vi "24.Evd.9_AskEfarmog.vi"() -> ()   [LabVIEW 2020]
uses:
  <vilib>/Native 3D Graph/xcontrol/3DPC_SurfacePlot.xctl
  <vilib>/measure/NI_MABase.lvlib
panel:
  in  "stop 3":bool
  out "Waveform Chart":waveform(dbl)[](graph)
  in  "Clear":bool
  in  "Boolean":bool
  in  "Boolean 2":bool
  in  "Boolean 3":bool
  in  "OK Button 4":bool
  in  "Frequency":dbl
  in  "Amplitude":dbl
  in  "stop 2":bool
  out "Waveform Graph":dbl[][](array[numeric])
  out "3D Graph":refnum<class "Base Datatype.lvclass">[](xcontrol)
  in  "OK Button 3":bool
  in  "Digital Data 2":digitaldata
  out "output waveform 2":digitalwaveform(waveform)={"t0"=timestamp(0 s since 1904-01-01), "dt"=1.0, "Y"={"transitions"=[], "data"=[]}}
  in  "stop":bool
  in  "OK Button 2":bool
  out "Digital Waveform Graph 3":digitalwaveform(graph)
  out "Digital Waveform Graph":digitalwaveform(graph)
  out "Sine Wave":waveform(dbl)[](graph)
  out "XY Graph":cluster{i32[], dbl[]}(graph)
  out "Random Array":dbl[](array[numeric])
  out "Waveform":waveform(dbl)[](graph)
  out "output waveform":digitalwaveform(waveform)={"t0"=timestamp(0 s since 1904-01-01), "dt"=1.0, "Y"={"transitions"=[], "data"=[]}}
  in  "Digital Data":digitaldata
  out "Mixed Signal Graph":T1(graph)
  out "Digital Waveform Graph 2":digitalwaveform(graph)
  in  "OK Button":bool
  # "11,33"
  # "11,35"
  # "11,39"
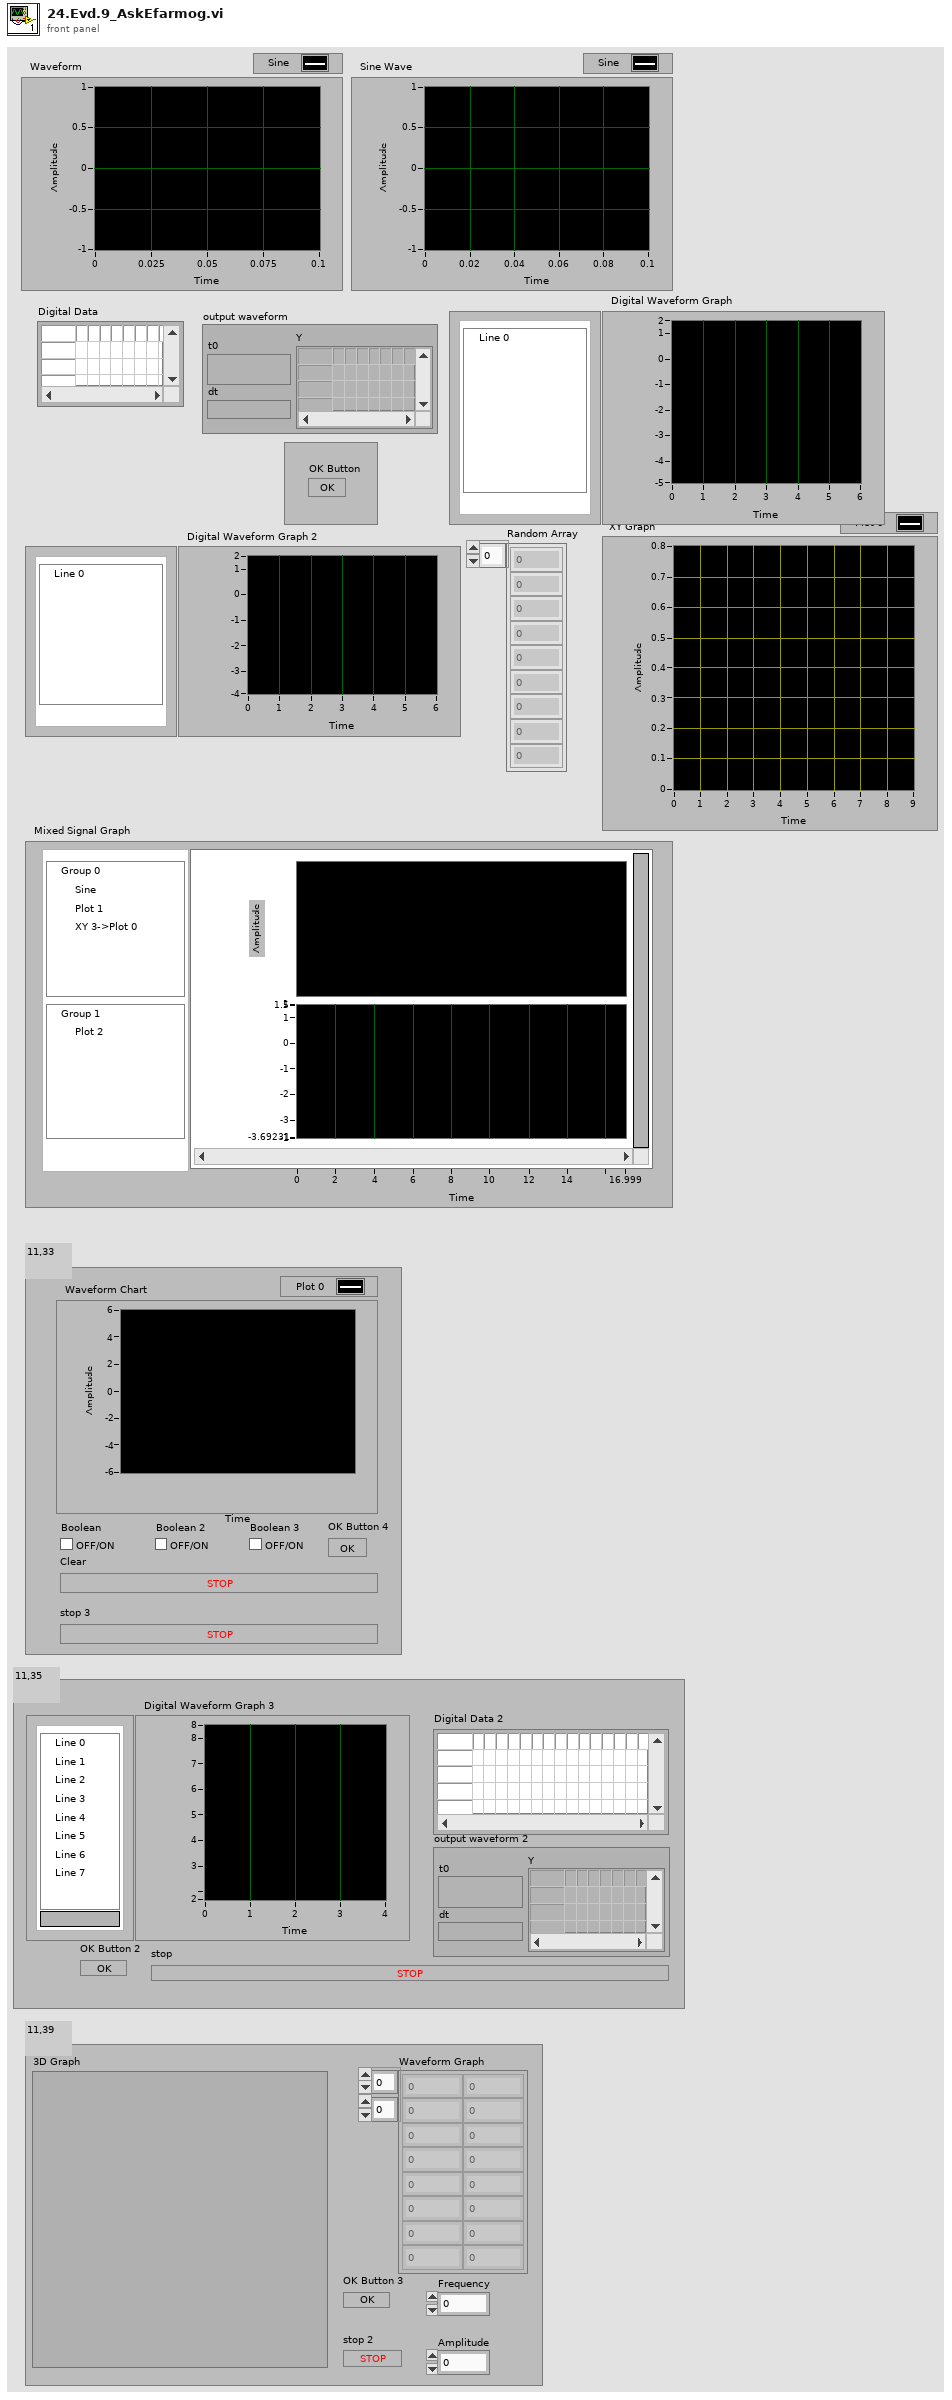
[diagram p1: front panel]
types:
  T1 = cluster{"Array of Waveform":waveform(dbl)[], dbl[], digitalwaveform, cluster{i32[], dbl[]}}
  T2 = typedef "imagedata.ctl" = cluster{"image type":i32, "image depth":i32, "image":u8[], "mask":u8[], "colors":u32[], "Rectangle":cluster{"left":i16, "top":i16, "right":i16, "bottom":i16}}
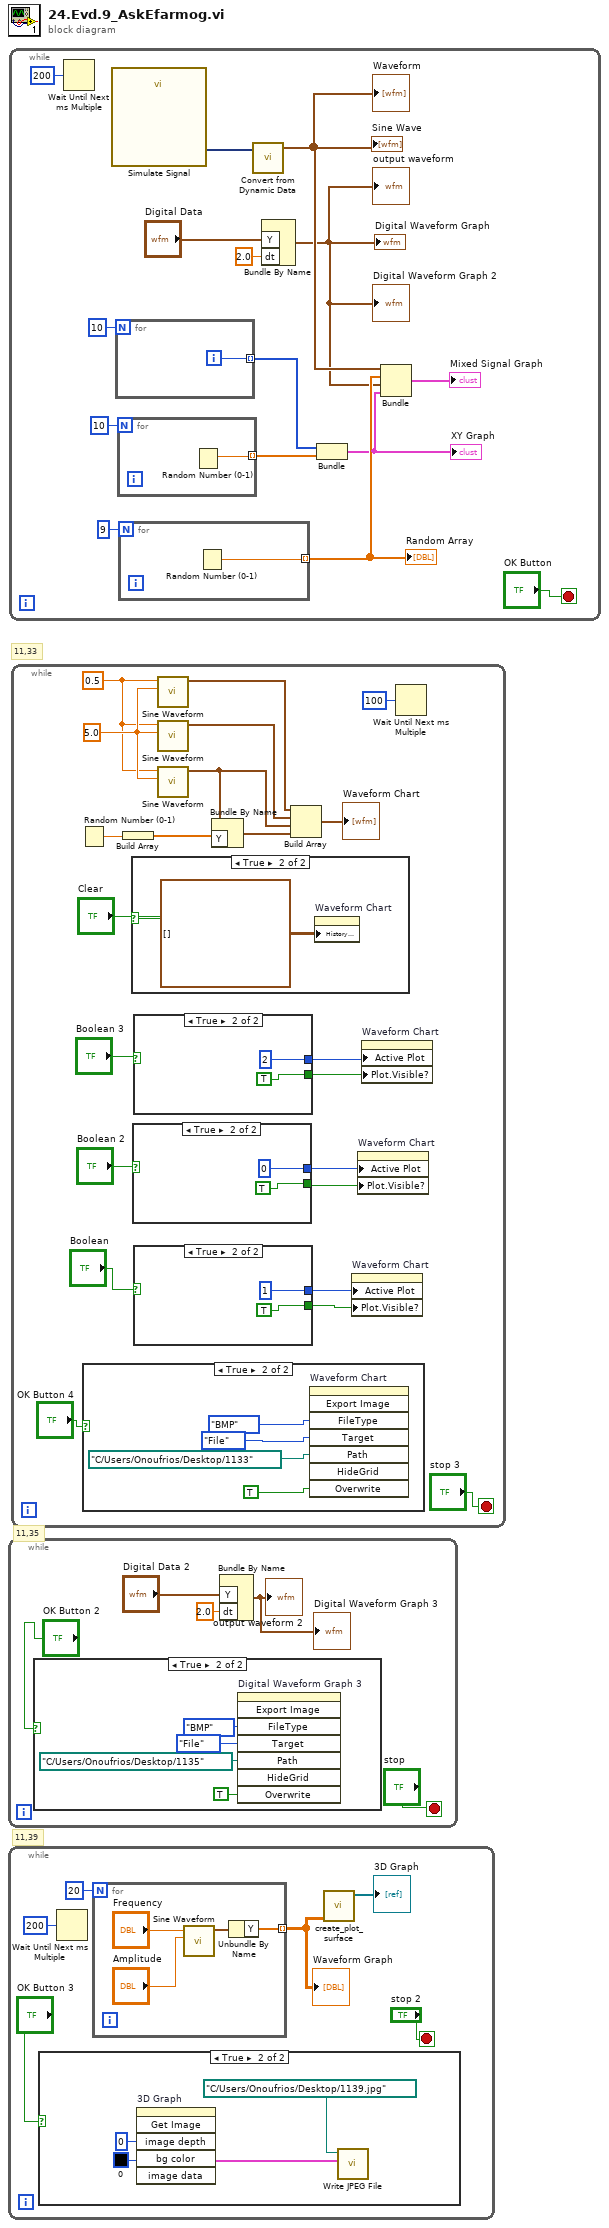
[diagram p0: block diagram]
diagram:
  # "11,33"
  # "11,35"
  # "11,39"
  n1 = while {
    stop <- "stop" stop-if-true
    n2 = case shown="True" "OK Button 2" {
      frame False {
      }
      frame True {
        n3 = invoke on="Digital Waveform Graph 3" class="DigitalGraph (strict)" method="Export Image"("FileType"=enum32{"BMP", "EPS", "EMF", "PICT"}."BMP" ("File Type"), "Target"=enum32{"File", "Clipboard"}."File", "Path"=path "C:/Users/Onoufrios/Desktop/1135", "Overwrite"=TRUE ("Always Overwrite")) -> ()  [unwired: 4 in, 8 out]
      }
    }
    n4 = Bundle By Name("Y"="Digital Data 2", "dt"=2.0) -> (→"output waveform 2" →"Digital Waveform Graph 3":digitalwaveform)  [unwired: 1 in]
  }
  n5 = while {
    stop <- "stop 2" stop-if-true
    n6 = case shown="True" "OK Button 3" {
      frame False {
      }
      frame True {
        n7 = invoke on="3D Graph" class="LabVIEW 3D Graph (strict)" method="Get Image"("image depth"=0 ("Image Depth"), "bg color"=u32 0 ("Background Color")) -> ("image data"=w17:T2)  [unwired: 4 in, 5 out]
        n8 = call <vilib>:"Write JPEG File.vi"("image data"=w17, "path to JPEG file"=path "C:/Users/Onoufrios/Desktop/1139.jpg" ("Path")) -> ()  [unwired: 8 in, 2 out]
      }
    }
    n9 = Wait Until Next ms Multiple(millisecond multiple=u32 200) -> ()  [unwired: 1 out]
    n10 = for {
      N: 20 -> [_]
      tunnel: [w20] -> w11 mode=indexing
      n11 = call <vilib>:"Sine Waveform.vi"("amplitude"="Amplitude", "frequency"="Frequency") -> ("signal out"=w21:waveform(dbl))  [unwired: 8 in, 1 out]
      n12 = Unbundle By Name(w21) -> ("Y"=w20:dbl[])
    }
    "Waveform Graph" <- w11
    n13 = call <vilib>:"create_plot_surface.vi"("z matrix"=w11) -> ("plots out"=→"3D Graph":refnum<class "Base Datatype.lvclass">[])  [unwired: 5 in, 5 out]
  }
  n14 = while {
    stop <- "OK Button" stop-if-true
    n15 = Wait Until Next ms Multiple(millisecond multiple=u32 200) -> ()  [unwired: 1 out]
    n16 = call "Simulate Signal"() -> ("Sine"=w29:dynamicdata)  [unwired: 14 in, 1 out]
    n17 = for {
      N: 10 -> [_]
      tunnel: [w41] -> w33 mode=indexing
      i -> [w41]
    }
    n18 = for {
      N: 10 -> [_]
      tunnel: [w40] -> w24 mode=indexing
      n19 = Random Number (0-1)() -> (number: 0 to 1=w40:dbl)
    }
    n20 = for {
      N: 9 -> [_]
      tunnel: [w39] -> w31 mode=indexing
      n21 = Random Number (0-1)() -> (number: 0 to 1=w39:dbl)
    }
    "Random Array" <- w31
    n22 = call "Convert from Dynamic Data"("Dynamic Data Type"=w29) -> ("Array of Waveform"=w28:waveform(dbl)[])  [unwired: 3 in]
    "Waveform" <- w28
    "Sine Wave" <- w28
    n23 = Bundle By Name("Y"="Digital Data", "dt"=2.0) -> (w27:digitalwaveform)  [unwired: 1 in]
    "output waveform" <- w27
    "Digital Waveform Graph 2" <- w27
    "Digital Waveform Graph" <- w27
    n24 = Bundle(w33, w24) -> (w26:cluster{i32[], dbl[]})  [unwired: 1 in]
    "XY Graph" <- w26
    n25 = Bundle("Array of Waveform"=w28, w31, w27, w26) -> (→"Mixed Signal Graph":T1)  [unwired: 1 in]
  }
  n26 = while {
    stop <- "stop 3" stop-if-true
    w63 = 5.0 ("amplitude")
    w62 = 0.5 ("frequency")
    n27 = Random Number (0-1)() -> (number: 0 to 1=w61:dbl)
    n28 = case shown="True" "OK Button 4" {
      frame False {
      }
      frame True {
        n29 = invoke on="Waveform Chart" class="WFChart (strict)" method="Export Image"("FileType"=enum32{"BMP", "EPS", "EMF", "PICT"}."BMP" ("File Type"), "Target"=enum32{"File", "Clipboard"}."File", "Path"=path "C:/Users/Onoufrios/Desktop/1133", "Overwrite"=TRUE ("Always Overwrite")) -> ()  [unwired: 4 in, 8 out]
      }
    }
    n30 = Build Array(w61) -> (w60:dbl[])
    n31 = case shown="True" "Clear" {
      frame False {
      }
      frame True {
        n32 = property on="Waveform Chart" class="WFChart (strict)"("History Data"=waveform(dbl)[][] []) -> ()  [unwired: 2 in, 2 out]
      }
    }
    n33 = case shown="True" "Boolean 2" {
      tunnel: [_ u32 0 ("Active Plot")] -> w49
      tunnel: [_ TRUE ("Plot.Visible")] -> w48
      frame False {
      }
      frame True {
      }
    }
    n34 = case shown="True" "Boolean 3" {
      tunnel: [_ u32 2 ("Active Plot")] -> w51
      tunnel: [_ TRUE ("Plot.Visible")] -> w50
      frame False {
      }
      frame True {
      }
    }
    n35 = case shown="True" "Boolean" {
      tunnel: [_ u32 1 ("Active Plot")] -> w47
      tunnel: [_ TRUE ("Plot.Visible")] -> w46
      frame False {
      }
      frame True {
      }
    }
    n36 = call <vilib>:"Sine Waveform.vi"("amplitude"=w63, "frequency"=w62) -> ("signal out"=w56:waveform(dbl))  [unwired: 8 in, 1 out]
    n37 = call <vilib>:"Sine Waveform.vi"("amplitude"=w63, "frequency"=w62) -> ("signal out"=w57:waveform(dbl))  [unwired: 8 in, 1 out]
    n38 = call <vilib>:"Sine Waveform.vi"("amplitude"=w63, "frequency"=w62) -> ("signal out"=w58:waveform(dbl))  [unwired: 8 in, 1 out]
    n39 = Bundle By Name(cluster=w58, "Y"=w60) -> (w59:waveform(dbl))
    n40 = Build Array(w56, w57, w58, w59) -> (→"Waveform Chart":waveform(dbl)[])
    n41 = property on="Waveform Chart" class="WFChart (strict)"("Active Plot"=w47, "Plot.Visible?"=w46) -> ()  [unwired: 2 in, 2 out]
    n42 = property on="Waveform Chart" class="WFChart (strict)"("Active Plot"=w49, "Plot.Visible?"=w48) -> ()  [unwired: 2 in, 2 out]
    n43 = property on="Waveform Chart" class="WFChart (strict)"("Active Plot"=w51, "Plot.Visible?"=w50) -> ()  [unwired: 2 in, 2 out]
    n44 = Wait Until Next ms Multiple(millisecond multiple=u32 100) -> ()  [unwired: 1 out]
  }
